vi "Update Entity Details.vi"(7 "entity type":T1, 8 "error in (no error)":errorcluster, 9 "status":string, 10 "enqueuer":refnum<class "Message Enqueuer.lvclass">, 11 "Coffee Shop in":refnum<class "Coffee Shop.lvclass">) -> (0 "error out":errorcluster, 3 "Coffee Shop out":refnum<class "Coffee Shop.lvclass">)   [LabVIEW 2023, in "Coffee Shop.lvlib" / "Coffee Shop.lvclass"]
doc: "Update the status internal to the entity table, then update the display of the table on the UI."
uses:
  Coffee Shop.lvclass
  <vilib>/ActorFramework/Message Enqueuer/Message Enqueuer.lvclass
  Entity Types.ctl
  Coffee Shop.lvclass/Coffee Shop.ctl
  Entity Table/Entity Table.lvclass
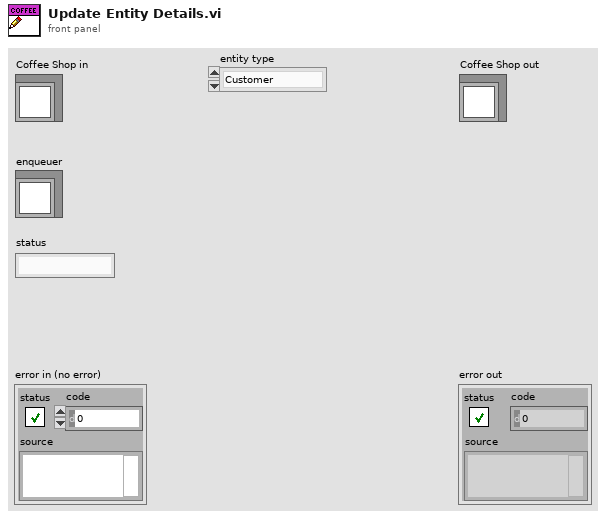
[diagram p1: front panel]
types:
  T1 = typedef "Coffee Shop.lvlib/Coffee Shop.lvclass/Entity Types.ctl" = enum16{"Customer", "Cashier", "Barista"}
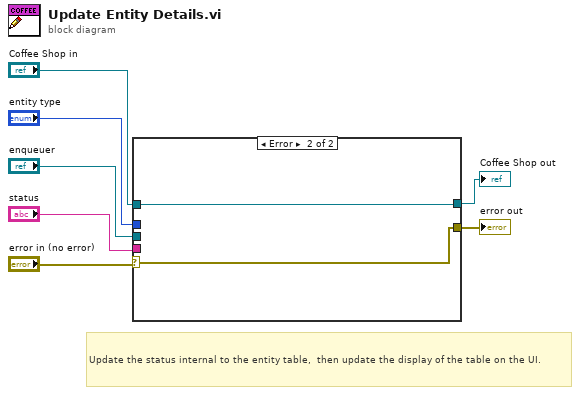
[diagram p0: block diagram]
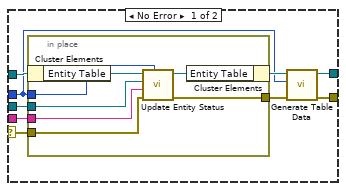
[diagram p2: hidden frame]
diagram:
  # "Update the status internal to the entity table,  then update the display of the table on the UI."
  n1 = case shown="Error" "error in (no error)" {
    selector: "error in (no error)" -> [w12 w25]
    tunnel: [w15 w25] -> w6
    tunnel: [w13 w24] -> w4
    tunnel: "Coffee Shop in" -> [w16 w24]
    tunnel: "entity type" -> [w8 _]
    tunnel: "enqueuer" -> [w10 _]
    tunnel: "status" -> [w9 _]
    frame No Error {
      n2 = in-place {
        in-place-border: w8 -> [w21]
        in-place-border: w12 -> [w20]
        in-place-border: [w19] -> w11
        in-place-border: w10 -> [w18]
        in-place-border: w9 -> [w17]
        n3 = in-place-cluster #1(w16) -> ("Entity Table"=w23:refnum<class "Entity Table.lvclass">)
        n4 = call "Update Entity Status.vi"("entity type"=w21, "error in (no error)"=w20, "Status"=w17, "Enqueuer"=w18, "entities in"=w23) -> ("error out"=w19:errorcluster, "entities out"=w22:refnum<class "Entity Table.lvclass">)  [unwired: 5 in]
        n5 = in-place-cluster #1("Entity Table"=w22) -> (w14:refnum<class "Coffee Shop.lvclass">)
      }
      n6 = call-dynamic "Generate Table Data.vi"("error in (no error)"=w11, "Entity Type"=w8, "Coffee Shop in"=w14) -> ("error out"=w15:errorcluster, "Coffee Shop out"=w13:refnum<class "Coffee Shop.lvclass">)  [unwired: 7 in]
    }
    frame Error {
    }
  }
  "error out" <- w6
  "Coffee Shop out" <- w4
